vi "TestVI.vi"(6 "Numeric 2":dbl, 8 "error in (no error)":errorcluster, 9 "Boolean 2":bool, 10 "Numeric":dbl, 11 "Boolean":bool) -> (0 "error out":errorcluster, 1 "Numeric out 2":dbl, 2 "Numeric out":dbl, 3 "Boolean out":bool)   [LabVIEW 2020]
panel:
  in  "Switch":bool
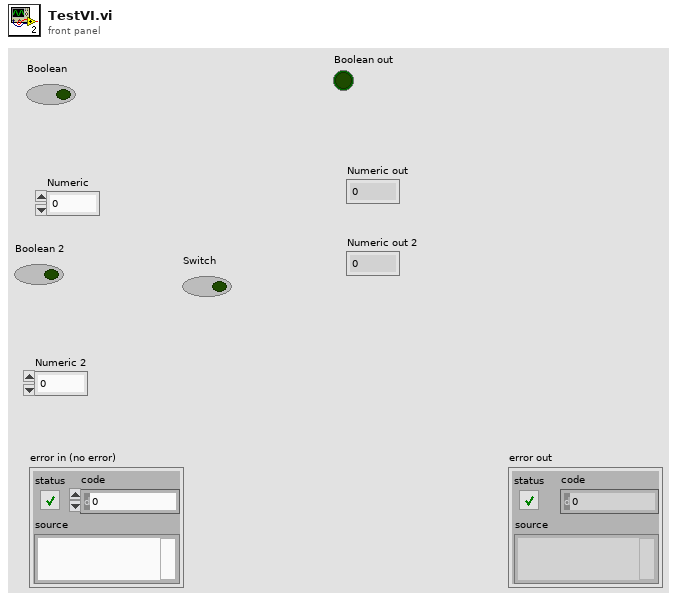
[diagram p1: front panel]
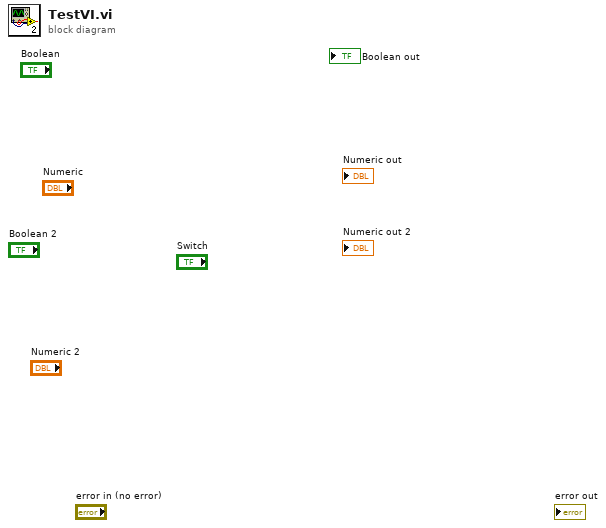
[diagram p0: block diagram]
diagram:
